vi "Boonton7200_Shutdown.vi"(7 "GPIB Address String":string, 8 "Error In":errorcluster) -> (0 "Error Out":errorcluster)   [LabVIEW 2015, in "Boonton7200.lvlib"]
uses:
  Boonton7200.lvlib
  Boonton7200_IEEE-488_Bus_Mnemonics.ctl
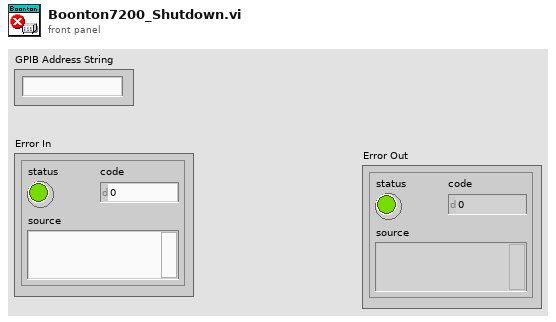
[diagram p1: front panel]
types:
  T1 = typedef "Boonton7200_IEEE-488_Bus_Mnemonics.ctl" = string
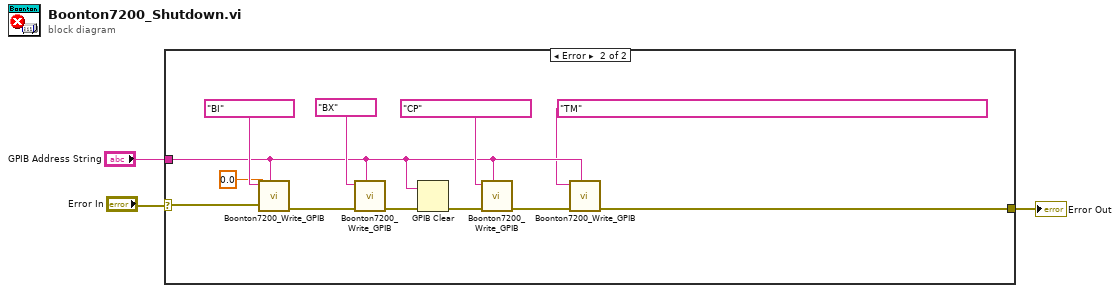
[diagram p0: block diagram]
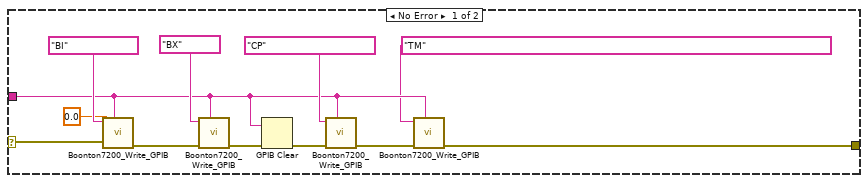
[diagram p2: hidden frame]
diagram:
  n1 = case shown="Error" "Error In" {
    selector: "Error In" -> [w5 w17]
    tunnel: "GPIB Address String" -> [w7 w19]
    tunnel: [w4 w16] -> w1
    frame No Error {
      n2 = call "Boonton7200_Write_GPIB.vi"("GPIB Address String"=w7, "Error In"=w5, "Data Value"=sgl 0.0, "IEEE-488 Bus Mnemonics"=T1 "BI") -> ("Error Out"=w13:errorcluster)  [unwired: 7 in]
      n3 = call "Boonton7200_Write_GPIB.vi"("GPIB Address String"=w7, "Error In"=w13, "IEEE-488 Bus Mnemonics"=T1 "BX") -> ("Error Out"=w14:errorcluster)  [unwired: 8 in]
      n4 = GPIB Clear(2:w14, 3:w7) -> (0:w10:errorcluster)  [unwired: 1 out]
      n5 = call "Boonton7200_Write_GPIB.vi"("GPIB Address String"=w7, "Error In"=w10, "IEEE-488 Bus Mnemonics"=T1 "CP") -> ("Error Out"=w9:errorcluster)  [unwired: 8 in]
      n6 = call "Boonton7200_Write_GPIB.vi"("GPIB Address String"=w7, "Error In"=w9, "IEEE-488 Bus Mnemonics"=T1 "TM") -> ("Error Out"=w4:errorcluster)  [unwired: 8 in]
    }
    frame Error {
      n7 = call "Boonton7200_Write_GPIB.vi"("GPIB Address String"=w19, "Error In"=w17, "Data Value"=sgl 0.0, "IEEE-488 Bus Mnemonics"=T1 "BI") -> ("Error Out"=w25:errorcluster)  [unwired: 7 in]
      n8 = call "Boonton7200_Write_GPIB.vi"("GPIB Address String"=w19, "Error In"=w25, "IEEE-488 Bus Mnemonics"=T1 "BX") -> ("Error Out"=w26:errorcluster)  [unwired: 8 in]
      n9 = GPIB Clear(2:w26, 3:w19) -> (0:w22:errorcluster)  [unwired: 1 out]
      n10 = call "Boonton7200_Write_GPIB.vi"("GPIB Address String"=w19, "Error In"=w22, "IEEE-488 Bus Mnemonics"=T1 "CP") -> ("Error Out"=w21:errorcluster)  [unwired: 8 in]
      n11 = call "Boonton7200_Write_GPIB.vi"("GPIB Address String"=w19, "Error In"=w21, "IEEE-488 Bus Mnemonics"=T1 "TM") -> ("Error Out"=w16:errorcluster)  [unwired: 8 in]
    }
  }
  "Error Out" <- w1
